vi "Create from Session.vi"(8 "Error In":errorcluster, 11 "Session":refnum<class "Session.lvclass">) -> (0 "Error Out":errorcluster, 3 "Known Hosts":refnum<class "Known Hosts.lvclass">)   [LabVIEW 2018, in "Toolkit.lvlib" / "Known Hosts.lvclass"]
doc: "Creates a new Known Hosts object from a Session object."
uses:
  Known Hosts.lvclass
  Session/Session.lvclass
  Session/Session.lvclass/Session.ctl
  SSH/SSH.lvclass/SSH.ctl
  Known Hosts.lvclass/Known Hosts.ctl
  Toolkit.lvlib
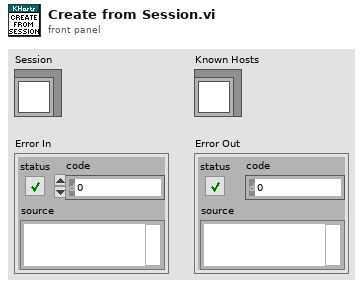
[diagram p1: front panel]
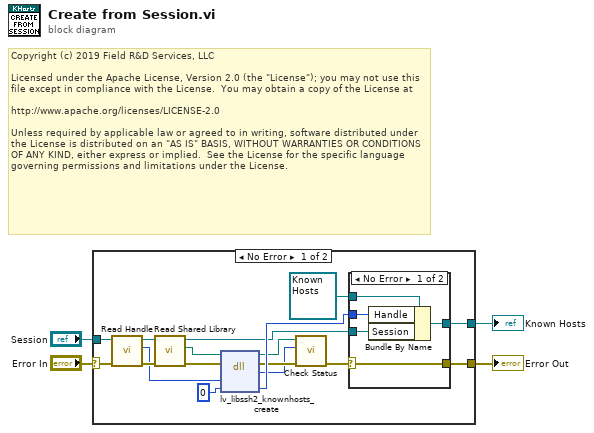
[diagram p0: block diagram]
diagram:
  # "Copyright (c) 2019 Field R&D Services, LLC\n\nLicensed under the Apache License, Version 2.0 (the \"License\"); you may not use this file except in compliance with the License.  You may obtain a copy of the License at\n\nhttp://www.apache.org/licenses/LICENSE-2.0\n\nUnless required by applicable law or agreed to in writing, software distributed under the License is distributed on an \"AS IS\" BASIS, WITHOUT WARRANTIES OR CONDITIONS OF ANY KIND, either express or implied.  See the License for the specific language governing permissions and limitations under the License."
  n1 = case shown="No Error" "Error In" {
    selector: "Error In" -> [w19 w29]
    tunnel: [w7 w29] -> w3
    tunnel: "Session" -> [w20 _]
    tunnel: [w21 _] -> w1
    frame No Error {
      n2 = call "Read Handle.vi"("Error In"=w19, "Session In"=w20) -> ("Erorr Out"=w17:errorcluster, "Handle"=w14:u64, "Session Out"=w18:refnum<class "Session.lvclass">)  [unwired: 7 in]
      n3 = call "Read Shared Library.vi"("Error In"=w17, "Session In"=w18) -> ("Erorr Out"=w16:errorcluster, "libssh2lv Shared Library"=w15:path, "Session Out"=w6:refnum<class "Session.lvclass">)  [unwired: 7 in]
      n4 = dll-call lib="D:/Users/cfield/Code/Field R&D Services/SSH/LV-LIBSSH2/LabVIEW/trunk/src/Toolkit/Support/lv-libssh2.*" fn="lv_libssh2_knownhosts_create"(path in=w15, error in=w16, "session"=w14, "handle"=u64 0) -> (path out=w9:path, error out=w11:errorcluster, "status"=w10:i32, "handle"=w12:u64)  [unwired: 2 in]
      n5 = call "Check Status.vi"("Error In"=w11, "Status"=w10, "libssh2lv Shared Library In"=w9) -> ("Error Out"=w8:errorcluster)  [unwired: 7 in, 1 out]
      n6 = case shown="No Error" w8 {
        selector: w8 -> [w24 w28]
        tunnel: [w26 w27] -> w21
        tunnel: w12 -> [w25 _]
        tunnel: [w24 w28] -> w7
        tunnel: w6 -> [w23 _]
        tunnel: refnum<class "Known Hosts.lvclass"> refnum ("LabSSH2.lvlib:KnownHosts.lvclass") -> [w22 w27]
        frame No Error {
          n7 = Bundle By Name(cluster=w22, "Handle"=w25, "Session"=w23) -> (w26:refnum<class "Known Hosts.lvclass">)
        }
        frame Error {
        }
      }
    }
    frame Error {
    }
  }
  "Error Out" <- w3
  "Known Hosts" <- w1
